vi "XY Plot Buffer.vi"(10 "Desired":dbl[](array[numeric]), 11 "Actual":dbl[](array[numeric])) -> (3 "Buffered Task Coordinates":cluster{dbl[], dbl[]}[](array[cluster]))   [LabVIEW 2018]
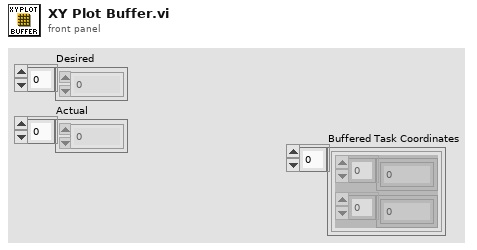
[diagram p1: front panel]
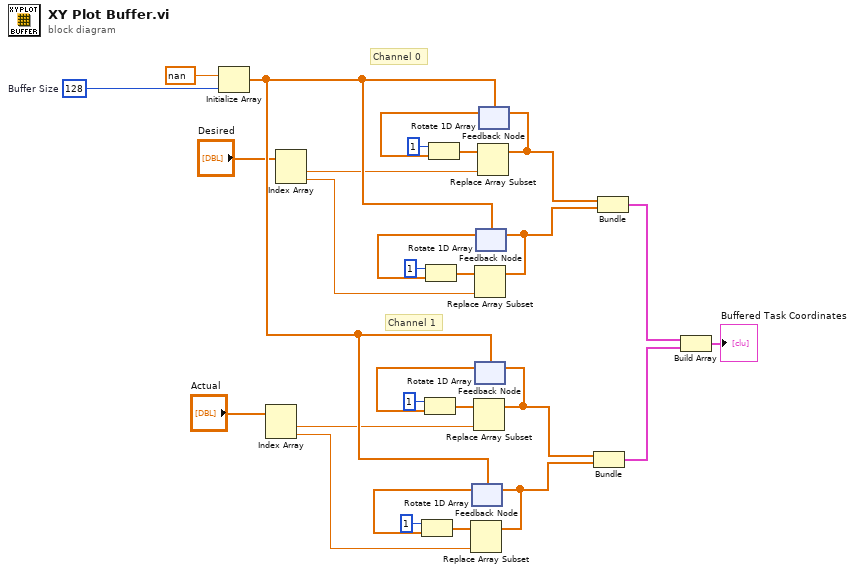
[diagram p0: block diagram]
diagram:
  w20 = 128  # Buffer Size
  # "Channel 1"
  # "Channel 0"
  n1 = Initialize Array(nan ("element"), w20) -> (w10:dbl[])
  n2 = Index Array(array="Actual") -> (element #1=w2:dbl, element #2=w1:dbl)  [unwired: 2 in]
  n3 = Index Array(array="Desired") -> (element #1=w6:dbl, element #2=w5:dbl)  [unwired: 2 in]
  n4 = feedback #1(w10) -> (w14:dbl[])
  n5 = Rotate 1D Array(1:w14, 2:1 ("n")) -> (0:w16:dbl[])
  n6 = Replace Array Subset(array=w16, new element=w1) -> (w18:dbl[])  [unwired: 1 in]
  n7 = feedback-in #1(w18) -> ()
  n8 = feedback #2(w10) -> (w13:dbl[])
  n9 = Rotate 1D Array(1:w13, 2:1 ("n")) -> (0:w11:dbl[])
  n10 = Replace Array Subset(array=w11, new element=w2) -> (w17:dbl[])  [unwired: 1 in]
  n11 = feedback-in #2(w17) -> ()
  n12 = feedback #3(w10) -> (w25:dbl[])
  n13 = Rotate 1D Array(1:w25, 2:1 ("n")) -> (0:w23:dbl[])
  n14 = Replace Array Subset(array=w23, new element=w5) -> (w21:dbl[])  [unwired: 1 in]
  n15 = feedback-in #3(w21) -> ()
  n16 = feedback #4(w10) -> (w26:dbl[])
  n17 = Rotate 1D Array(1:w26, 2:1 ("n")) -> (0:w28:dbl[])
  n18 = Replace Array Subset(array=w28, new element=w6) -> (w22:dbl[])  [unwired: 1 in]
  n19 = feedback-in #4(w22) -> ()
  n20 = Bundle(w17, w18) -> (w8:cluster{dbl[], dbl[]})  [unwired: 1 in]
  n21 = Bundle(w22, w21) -> (w9:cluster{dbl[], dbl[]})  [unwired: 1 in]
  n22 = Build Array(w9, w8) -> (→"Buffered Task Coordinates":cluster{dbl[], dbl[]}[])
